vi "Set Assertion Type.vi"(10 "Assertion Type":T1=enum."Pass", 11 "LUnit Test Case In":refnum<class "LUnit Test Case.lvclass">) -> (3 "LUnit Test Case Out":refnum<class "LUnit Test Case.lvclass">)   [LabVIEW 2020, in "LUnit Test Case.lvclass"]
uses:
  LUnit Test Case.lvclass
  Result Types/Assertion Result/Public/TypeDefs/Assertion Type.ctl
  LUnit Test Case.lvclass/LUnit Test Case.ctl
  Rewrite Project/Result/Result.lvlib
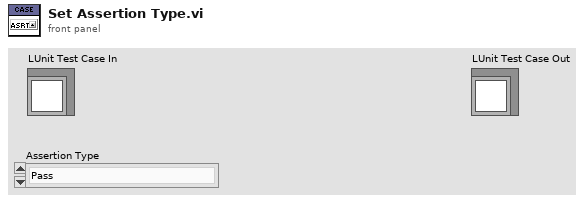
[diagram p1: front panel]
types:
  T1 = typedef "Result.lvlib/Assertion Type.ctl" = enum16{"None", "Pass", "Fail", "Skip", "Pass if Equal", "Fail if Equal", "Pass if Error", "Fail if Error", "Pass if", "Fail if"}
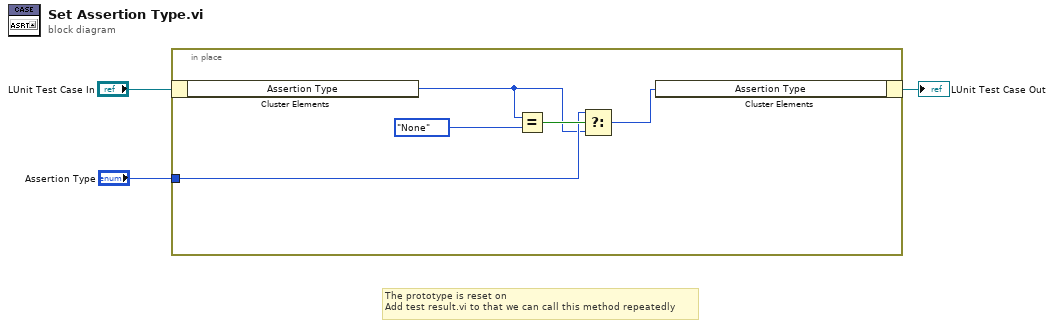
[diagram p0: block diagram]
diagram:
  # "The prototype is reset on \nAdd test result.vi to that we can call this method repeatedly"
  n1 = in-place {
    in-place-border: "Assertion Type" -> [w6]
    n2 = in-place-cluster #1("LUnit Test Case In") -> ("Assertion Type"=w5:T1)
    n3 = Equal?(x=w5, y=Assertion_Type."None" ("Assertion Type")) -> (x = y?=w7:bool)
    n4 = Select(t=w6, s=w7, f=w5) -> (s? t:f=w4:T1)
    n5 = in-place-cluster #1("Assertion Type"=w4) -> (→"LUnit Test Case Out":refnum<class "LUnit Test Case.lvclass">)
  }
